vi "DHE_SetDarkTime.vi"(6 "flush?":bool, 8 "error in (no error)":errorcluster, 9 "detstat":string, 10 "darktime":i32) -> (0 "error out":errorcluster)   [LabVIEW 2016]
uses:
  DBSHAND/private/vis/DatabaseHand_Element_Set(double).vi
panel:
  out "darktimeset":dbl
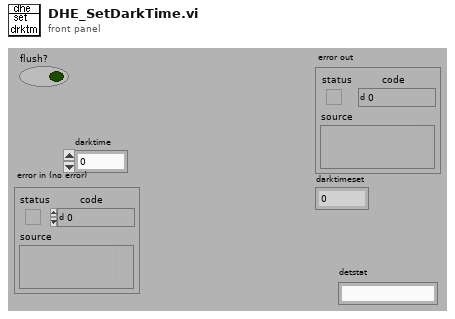
[diagram p1: front panel]
types:
  T1 = typedef "DatabaseHand_RefNum.ctl" = refnum<vi>
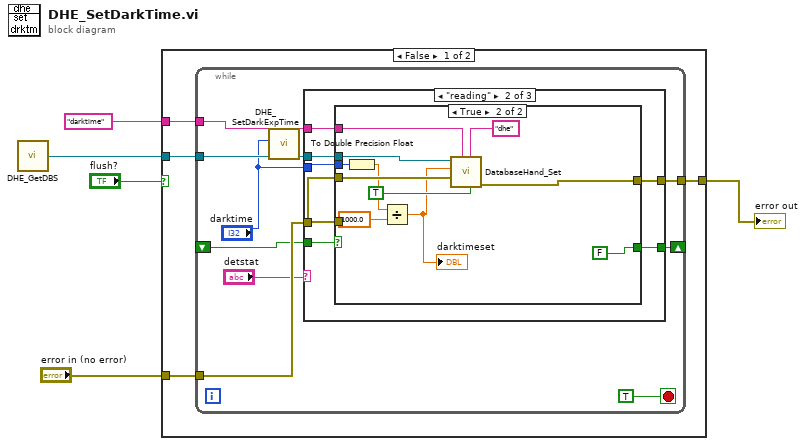
[diagram p0: block diagram]
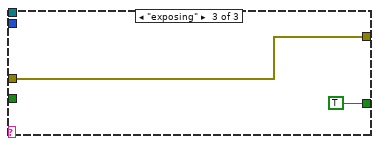
[diagram p4: hidden frame]
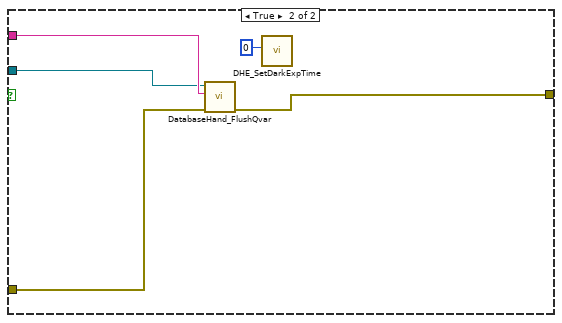
[diagram p5: hidden frame]
diagram:
  n1 = call "DHE_GetDBS.vi"() -> ("DHE_DBSRef"=w3:T1)  [unwired: 9 out]
  n2 = case shown="False" "flush?" {
    tunnel: "darktime" ("name") -> [w8 w47]
    tunnel: w3 -> [w9 w46]
    tunnel: "error in (no error)" -> [w7 w45]
    tunnel: [w6 w44] -> w1
    frame False {
      n3 = while {
        tunnel: w9 -> [w18]
        tunnel: w8 -> [w17]
        tunnel: w7 -> [w16]
        tunnel: [w15] -> w6
        shift-right: [w12] -> _
        shift-left: _ -> [w11]
        stop <- TRUE stop-if-true
        n4 = call "DHE_SetDarkExpTime.vi"("DarkExpTime"="darktime") -> ()  [unwired: 11 out]
        n5 = case shown="\"reading\"" "detstat" {
          tunnel: w18 -> [_ w27 _]
          tunnel: w17 -> [_ w26 _]
          tunnel: "darktime" -> [_ w25 _]
          tunnel: w16 -> [w20 w21 w41]
          tunnel: [w20 w24 w41] -> w15
          tunnel: [w19 w23 TRUE ("enqueue? (F)")] -> w12
          tunnel: w11 -> [w19 w22 _]
          frame Default {
          }
          frame "reading" {
            n6 = case shown="True" w22 {
              selector: w22 -> [w29 _]
              tunnel: w27 -> [_ w39]
              tunnel: w26 -> [_ w38]
              tunnel: w25 -> [_ w33]
              tunnel: w21 -> [_ w36]
              tunnel: [w28 w35] -> w24
              tunnel: [w29 FALSE ("enqueue? (F)")] -> w23
              tunnel: w21 -> [w28 _]
              frame False {
              }
              frame True {
                n7 = To Double Precision Float(number=w33) -> (double precision float=w31:dbl)
                n8 = Divide(x=w31, y=1000.0) -> (x/y=w32:dbl)
                "darktimeset" <- w32
                n9 = call-poly "DatabaseHand_Set.vi"("enqueue? (F)"=TRUE, "group"="dhe", "name"=w38, "error in (no error)"=w36, "value"=w32, "Database RefNum in"=w39) -> ("error out"=w35:errorcluster)  [unwired: 2 in, 3 out]
              }
            }
          }
          frame "exposing" {
          }
        }
      }
    }
    frame True {
      n10 = call "DatabaseHand_FlushQvar.vi"("error in (no error)"=w45, "name"=w47, "Database RefNum In"=w46) -> ("error out"=w44:errorcluster)  [unwired: 8 out]
      n11 = call "DHE_SetDarkExpTime.vi"("DarkExpTime"=u32 0) -> ()  [unwired: 11 out]
    }
  }
  "error out" <- w1
